vi "FTW-WEB-CreateWebServiceINI.vi"(0 "Output Directory":path, 1 "Default Document":string, 5 "Service Name":string, 7 "Request Handler Callback Filepaths":path[](array[path]), 9 "Routing Rules":T2(array[cluster]), 11 "error in":errorcluster, 12 "Static File Server Relative Filepath":string) -> (4 "INI filepath":path, 15 "error out":errorcluster)   [LabVIEW 2013]
uses:
  <vilib>/AppBuilder/AB_Classes/RESTful/AB_RESTful_HTTPMethodType.ctl
  <vilib>/AppBuilder/Engine/RESTful INI Generator/AB_RESTful_ServiceInfo.ctl
  <vilib>/AppBuilder/Engine/RESTful INI Generator/AB_RESTful_ServiceType.ctl
  <vilib>/AppBuilder/AB_Classes/RESTful/AB_RESTful_ServiceAttribute.ctl
  <vilib>/AppBuilder/AB_Classes/RESTful/AB_RESTful_ServiceAttributeType.ctl
  <vilib>/AppBuilder/AB_Classes/Source/RESTfulVI/Configure_RESTfulVI/AB_RESTful_Configuration.ctl
  <vilib>/AppBuilder/AB_Classes/Source/RESTfulVI/Configure_RESTfulVI/AB_RESTful_VIType.ctl
  <vilib>/AppBuilder/AB_Classes/Source/RESTfulVI/Configure_RESTfulVI/AB_RESTful_OutputType.ctl
  <vilib>/AppBuilder/AB_Classes/Source/RESTfulVI/Configure_RESTfulVI/AB_RESTful_OutputFormat.ctl
  <vilib>/AppBuilder/AB_Classes/RESTful/AB_RESTful_RoutingTemplate.ctl
  <vilib>/AppBuilder/AB_Classes/RESTful/AB_RESTful_RoutingType.ctl
panel:
  # "Inputs"
  # "Outputs"
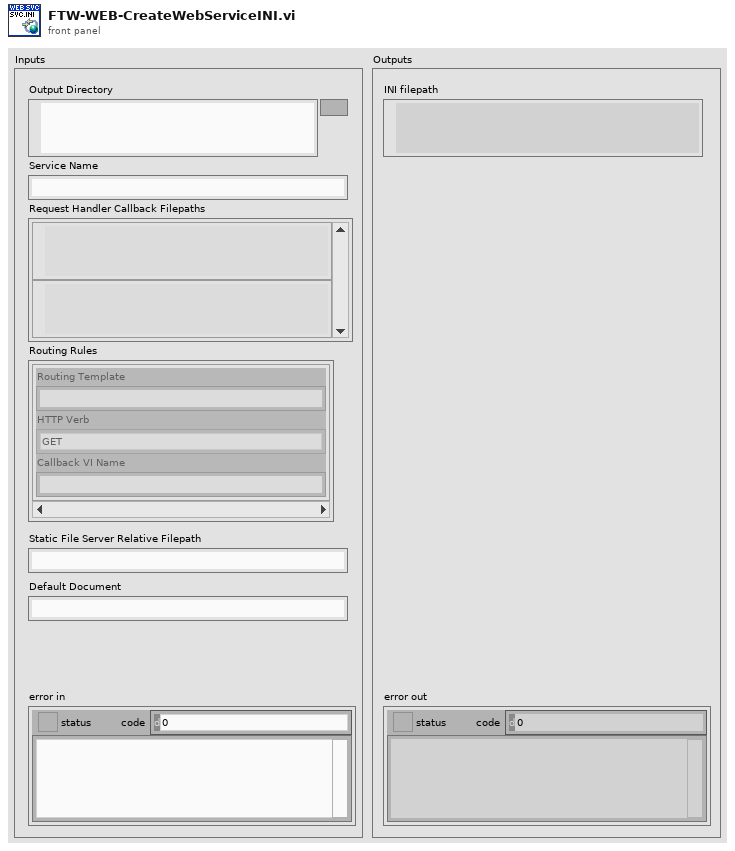
[diagram p1: front panel]
types:
  T1 = typedef "AB_RESTful_HTTPMethodType.ctl" = enum32{"GET", "POST", "PUT", "DELETE"}
  T2 = cluster{"Routing Template":string, "HTTP Verb":T1, "Callback VI Name":string}[]
  T3 = typedef "AB_RESTful_ServiceType.ctl" = enum32{"RESTful", "SOAP"}
  T4 = typedef "AB_RESTful_ServiceInfo.ctl" = cluster{"Service Name":string, "Service Type":T3, "Web Service Library Path":path, "Server List":string[], "Debug":bool, "Service aliases":string[], "defaultStaticDoc":string, "defaultWebMethod":string, "Standalone":bool, "Service attributes":T5[]}
  T5 = typedef "AB_RESTful_ServiceAttribute.ctl" = cluster{"Name":string, "Service Attribute Type":T6, "Value":string}
  T6 = typedef "AB_RESTful_ServiceAttributeType.ctl" = enum32{"String", "Path"}
  T7 = typedef "AB_RESTful_RoutingType.ctl" = enum32{"Method", "Static"}
  T8 = typedef "AB_RESTful_RoutingTemplate.ctl" = cluster{"Template":string, "Routing Type":T7, "HTTP Method Type":T1, "VIName":string, "Default String":string, "Require API key":bool, "Auth permissions":string[], "eng_Static Alias":string}
  T9 = typedef "AB_RESTful_Configuration.ctl" = cluster{"Service VI Type":T10, "Load VI at statup":bool, "Keep VI in memory":bool, "Output type":T11, "Output format":T12, "Use headers":bool, "Buffered":bool, "eng_Load VI by name":bool}
  T10 = typedef "AB_RESTful_VIType.ctl" = enum32{"Web Method", "Auxiliary", "eng_Internal", "eng_Content"}
  T11 = typedef "AB_RESTful_OutputType.ctl" = enum32{"Terminal", "Stream"}
  T12 = typedef "AB_RESTful_OutputFormat.ctl" = enum32{"XML", "Text", "HTML", "JSON"}
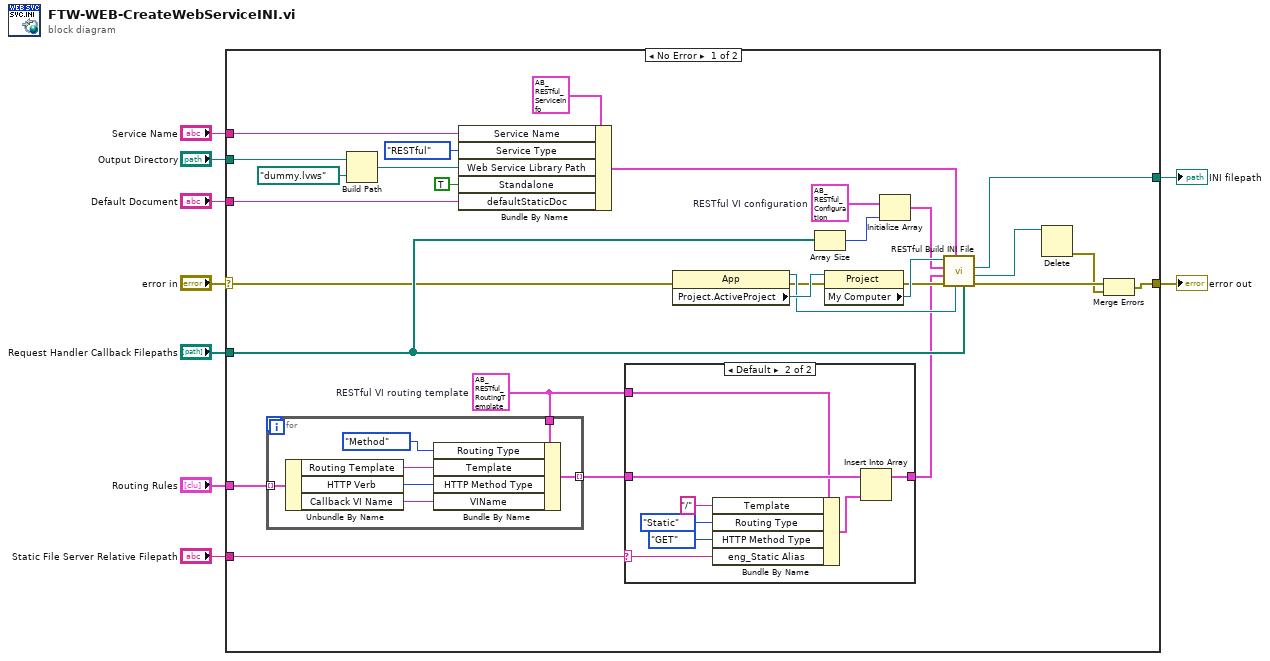
[diagram p0: block diagram]
diagram:
  n1 = case shown="No Error" "error in" {
    selector: "error in" -> [w18 w55]
    tunnel: [w34 _] -> w9
    tunnel: "Output Directory" -> [w17 _]
    tunnel: "Service Name" -> [w30 _]
    tunnel: "Request Handler Callback Filepaths" -> [w25 _]
    tunnel: [w21 w55] -> w5
    tunnel: "Routing Rules" -> [w19 _]
    tunnel: "Static File Server Relative Filepath" -> [w12 _]
    tunnel: "Default Document" -> [w10 _]
    frame No Error {
      w11 = T8 {"Template"="", "Routing Type"=enum."Static", "HTTP Method Type"=enum."GET", "VIName"="", "Default String"="", "Require API key"=FALSE, "Auth permissions"=[], "eng_Static Alias"=""}  # RESTful VI routing template
      w27 = T9 {"Service VI Type"=enum."Web Method", "Load VI at statup"=TRUE, "Keep VI in memory"=TRUE, "Output type"=enum."Stream", "Output format"=enum."Text", "Use headers"=TRUE, "Buffered"=TRUE, "eng_Load VI by name"=TRUE}  # RESTful VI configuration
      n2 = for {
        tunnel: w19 -> [w52] mode=indexing
        tunnel: [w53] -> w13 mode=indexing
        tunnel: w11 -> [w54]
        n3 = Unbundle By Name(w52) -> ("Routing Template"=w51:string, "HTTP Verb"=w50:T1, "Callback VI Name"=w49:string)
        n4 = Bundle By Name(cluster=w54, "Routing Type"=AB_RESTful_RoutingType."Method", "Template"=w51, "HTTP Method Type"=w50, "VIName"=w49) -> (w53:T8)
      }
      n5 = Build Path(base path=w17, name or relative path=path "dummy.lvws") -> (appended path=w16:path)
      n6 = Bundle By Name(cluster=T4 {"Service Name"="", "Service Type"=enum."RESTful", "Web Service Library Path"=path "", "Server List"=[], "Debug"=FALSE, "Service aliases"=[], "defaultStaticDoc"="", "defaultWebMethod"="", "Standalone"=FALSE, "Service attributes"=[]} ("RESTful VI service information"), "Service Name"=w30, "Service Type"=AB_RESTful_ServiceType."RESTful", "Web Service Library Path"=w16, "Standalone"=TRUE, "defaultStaticDoc"=w10) -> (w37:T4)
      n7 = case shown="Default" w12 {
        selector: w12 -> [_ w40]
        tunnel: [w39 w46] -> w14
        tunnel: w13 -> [w39 w47]
        tunnel: w11 -> [_ w45]
        frame "" {
        }
        frame Default {
          n8 = Bundle By Name(cluster=w45, "Template"="/", "Routing Type"=AB_RESTful_RoutingType."Static", "HTTP Method Type"=AB_RESTful_HTTPMethodType."GET", "eng_Static Alias"=w40) -> (w44:T8)
          n9 = Insert Into Array(array=w47, new element=w44) -> (w46:T8[])  [unwired: 1 in]
        }
      }
      n10 = property class="App"(error in=w18) -> (reference out=w32:refnum<vi>, error out=w28:errorcluster, "Project.ActiveProject"=w36:refnum<vi>)  [unwired: 1 in]
      n11 = Array Size(array=w25) -> (size(s)=w26:i32)
      n12 = property class="Project"(reference=w36, error in=w28) -> (error out=w29:errorcluster, "My Computer"=w35:refnum<vi>)  [unwired: 1 out]
      n13 = Initialize Array(w27, w26) -> (w24:T9[])
      n14 = call <vilib>:"RESTful Build INI File.vi"("relative VI paths"=w25, "buildContext"=w32, "RESTful VI service information"=w37, "error in (no error)"=w29, "Routing Templates"=w14, "VI Configurations"=w24, "target reference"=w35) -> ("error out"=w22:errorcluster, "XML filepath"=w23:path, "INI filepath"=w34:path)  [unwired: 1 in, 1 out]
      n15 = Delete(path (use dialog)=w23) -> (error out=w20:errorcluster)  [unwired: 4 in, 2 out]
      n16 = Merge Errors(w22, w20) -> (w21:errorcluster)
    }
    frame Error {
    }
  }
  "error out" <- w5
  "INI filepath" <- w9
